vi "Compass Bearing.vi"(0 "CurLatRad":dbl, 1 "CurLongRad":dbl, 2 "Latitude":dbl, 3 "Longitude":dbl, 4 "North or South":string, 5 "East or West":string) -> (20 "Compass":dbl(xcontrol))   [LabVIEW 2011]
uses:
  <vilib>/robotics/Controls/Compass Indicator/Compass Indicator.xctl
  <vilib>/express/express arith-compare/Formula/XNode/ExpressFormulaBlockNode.xnode
panel:
  out "Compass EW":string[](array[string])
  out "Compass NS":string[](array[string])
  out "Compass Long Array":dbl[](array[numeric]) format="%#_16g"
  out "Compass Lat Array":dbl[](array[numeric]) format="%#_16g"
  out "Compass Lat":dbl format="%#_16g"
  out "Compass Long":dbl format="%#_16g"
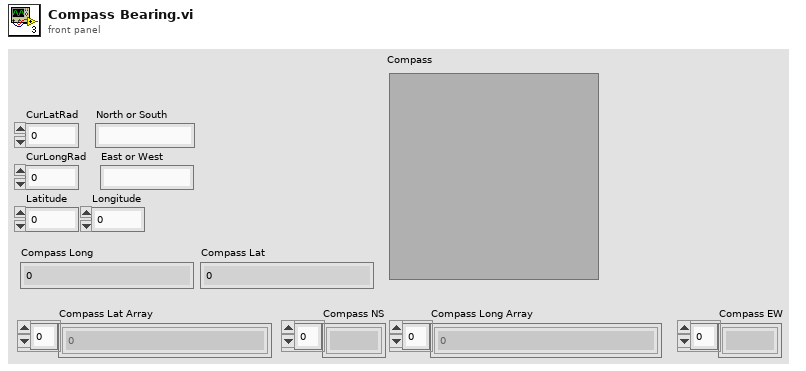
[diagram p1: front panel]
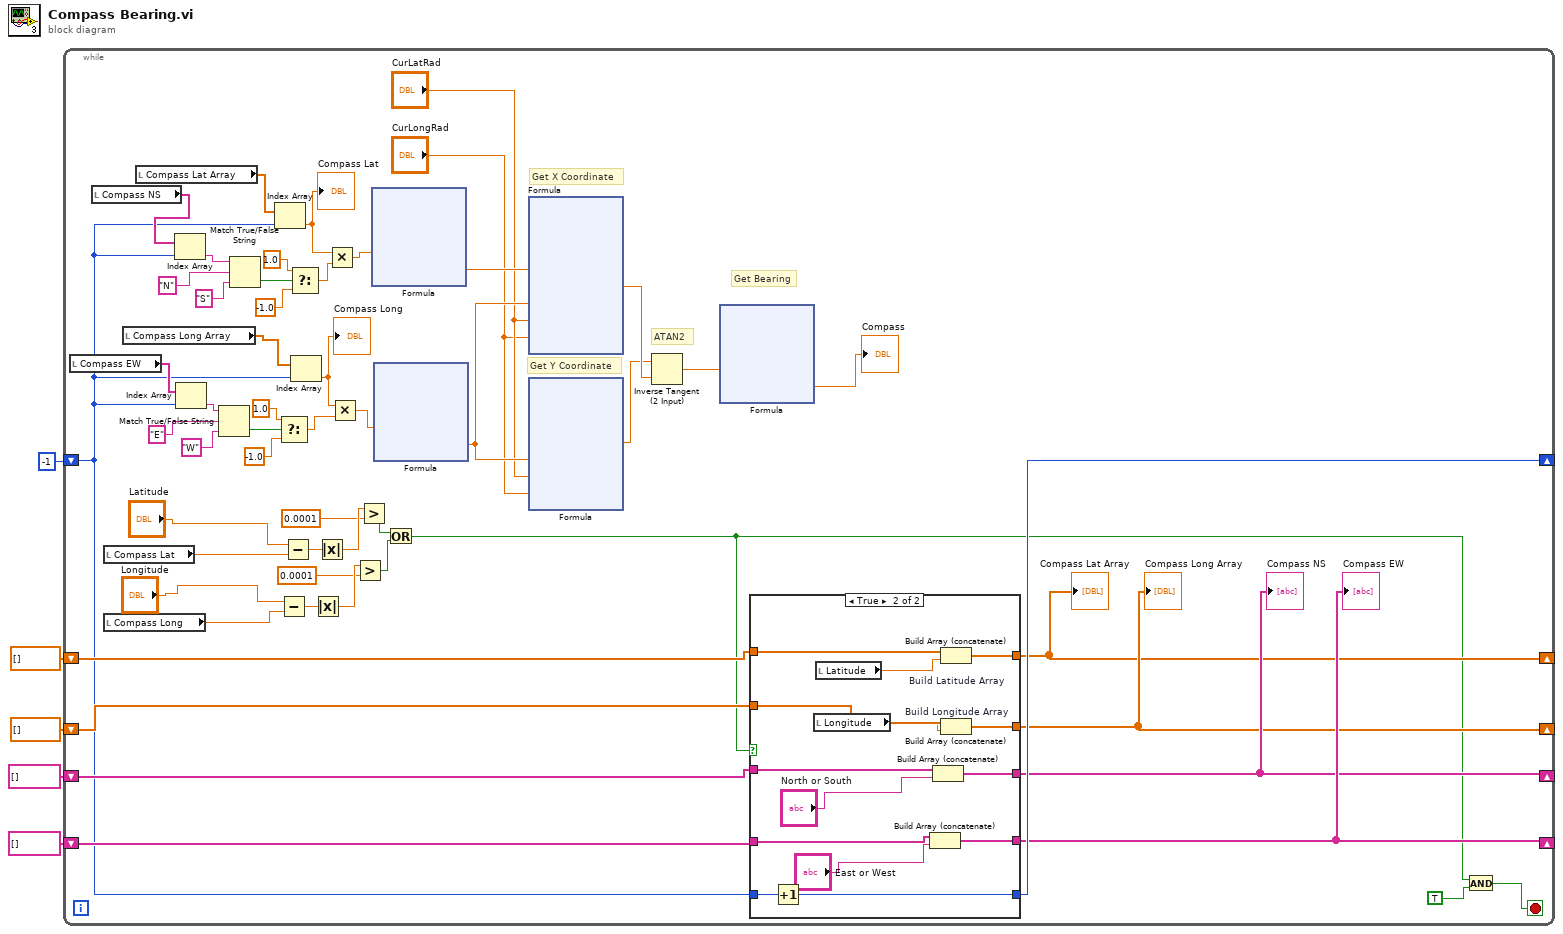
[diagram p0: block diagram]
diagram:
  n1 = while {
    shift-right: [w27] -> _
    shift-left: -1 -> [w14]
    shift-right: [w23] -> _
    shift-left: dbl[] [] -> [w19]
    shift-right: [w25] -> _
    shift-left: string[] [] -> [w21]
    shift-right: [w26] -> _
    shift-left: string[] [] -> [w22]
    shift-right: [w24] -> _
    shift-left: dbl[] [] -> [w20]
    stop <- w7 stop-if-true
    # "Get X Coordinate"
    # "Get Bearing"
    # "ATAN2"
    # "Get Y Coordinate"
    n2 = local read "Compass EW"() -> (w15:string[])
    n3 = local read "Compass NS"() -> (w17:string[])
    n4 = local read "Compass Lat"() -> (w36:dbl)
    n5 = local read "Compass Long"() -> (w37:dbl)
    n6 = local read "Compass Long Array"() -> (w16:dbl[])
    n7 = local read "Compass Lat Array"() -> (w18:dbl[])
    n8 = Index Array(array=w17, index=w14) -> (element=w43:string)
    n9 = Index Array(array=w15, index=w14) -> (element=w41:string)
    n10 = Match True/False String(2:"W" ("false string"), 3:"E" ("true string"), 4:w41) -> (0:w47:bool)  [unwired: 1 out]
    n11 = Match True/False String(2:"S" ("false string"), 3:"N" ("true string"), 4:w43) -> (0:w51:bool)  [unwired: 1 out]
    n12 = Index Array(array=w18, index=w14) -> (element=w44:dbl)
    "Compass Lat" <- w44
    n13 = Select(t=1.0, s=w47, f=-1.0) -> (s? t:f=w46:dbl)
    n14 = Subtract(x="Longitude", y=w37) -> (x-y=w32:dbl)
    n15 = Subtract(x="Latitude", y=w36) -> (x-y=w35:dbl)
    n16 = Select(t=1.0, s=w51, f=-1.0) -> (s? t:f=w45:dbl)
    n17 = Index Array(array=w16, index=w14) -> (element=w42:dbl)
    "Compass Long" <- w42
    n18 = Absolute Value(x=w32) -> (abs(x)=w31:dbl)
    n19 = Absolute Value(x=w35) -> (abs(x)=w34:dbl)
    n20 = Multiply(x=w44, y=w45) -> (x*y=w40:dbl)
    n21 = Multiply(x=w42, y=w46) -> (x*y=w39:dbl)
    n22 = Greater?(x=w31, y=0.0001 ("x")) -> (0:w28:bool)
    n23 = Greater?(x=w34, y=0.0001 ("x")) -> (0:w29:bool)
    n24 = xnode "Formula"("Dlat1"=w40) -> ("Result"=w56:dbl)  [unwired: 1 in, 1 out]
    n25 = xnode "Formula"("Dlong1"=w39) -> ("Result"=w57:dbl)  [unwired: 1 in, 1 out]
    n26 = Or(x=w29, y=w28) -> (x .or. y?=w6:bool)
    n27 = xnode "Formula"("PreLat"=w56, "PreLong"=w57, "CurLat"="CurLatRad", "CurLong"="CurLongRad") -> ("Result"=w59:dbl)  [unwired: 1 in, 1 out]
    n28 = xnode "Formula"("PreLong"=w57, "CurLat"="CurLatRad", "CurLong"="CurLongRad") -> ("Result"=w58:dbl)  [unwired: 1 in, 1 out]
    n29 = Inverse Tangent (2 Input)(1:w59, 2:w58) -> (0:w60:dbl)
    n30 = xnode "Formula"("rad"=w60) -> ("Result"=→"Compass":dbl)  [unwired: 1 in, 1 out]
    n31 = case shown="True" w6 {
      tunnel: w21 -> [w63 w79]
      tunnel: w22 -> [w62 w78]
      tunnel: w20 -> [w64 w77]
      tunnel: w19 -> [w65 w76]
      tunnel: [w62 w73] -> w26
      tunnel: [w63 w72] -> w25
      tunnel: [w64 w71] -> w24
      tunnel: [w65 w70] -> w23
      tunnel: w14 -> [w61 w69]
      tunnel: [w61 w68] -> w27
      frame False {
      }
      frame True {
        n32 = Increment(x=w69) -> (x+1=w68:i32)
        n33 = local read "Longitude"() -> (w74:dbl)
        n34 = local read "Latitude"() -> (w75:dbl)
        n35 = Build Array (concatenate)(w78, "East or West") -> (w73:string[])
        n36 = Build Array (concatenate)(w79, "North or South") -> (w72:string[])
        n37 = Build Array (concatenate) "Build Latitude Array"(w76, w75) -> (w70:dbl[])
        n38 = Build Array (concatenate) "Build Longitude Array"(w77, w74) -> (w71:dbl[])
      }
    }
    "Compass Lat Array" <- w23
    "Compass Long Array" <- w24
    "Compass NS" <- w25
    "Compass EW" <- w26
    n39 = And(x=w6, y=TRUE) -> (x .and. y?=w7:bool)
  }
